vi "PID dT.vi"(10 "Last Time":u32, 11 "Current Time":u32) -> (3 "Change in Time":u32)   [LabVIEW 2014]
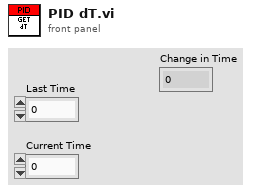
[diagram p1: front panel]
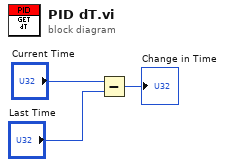
[diagram p0: block diagram]
diagram:
  n1 = Subtract(x="Current Time", y="Last Time") -> (x-y=→"Change in Time":u32)
